vi "opticPath2freq.vi"(1 "b":dbl, 2 "m":dbl, 3 "lamda (nm)":dbl, 4 "camino optico (nm)":dbl) -> (0 "freq":dbl)   [LabVIEW 2010]
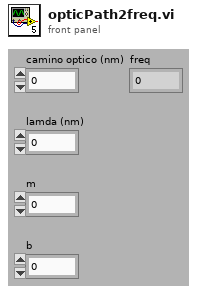
[diagram p1: front panel]
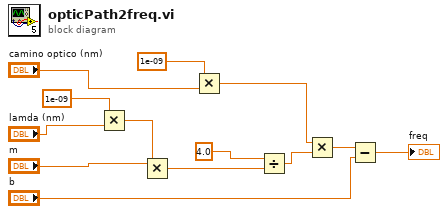
[diagram p0: block diagram]
diagram:
  n1 = Multiply(x=1e-09, y="lamda (nm)") -> (x*y=w5:dbl)
  n2 = Multiply(x="m", y=w5) -> (x*y=w11:dbl)
  n3 = Multiply(x=1e-09, y="camino optico (nm)") -> (x*y=w2:dbl)
  n4 = Divide(x=4.0, y=w11) -> (x/y=w7:dbl)
  n5 = Multiply(x=w2, y=w7) -> (x*y=w8:dbl)
  n6 = Subtract(x=w8, y="b") -> (x-y=→"freq":dbl)
